vi "GEA2 Log Filter.vi"(1 "DST to ignore":string, 2 "Only print Dst":string, 5 "Filter Data":bool, 7 "GEA2 Msg":T1 {"Command" format="%02x"; "Destination" format="%02x"; "Source" format="%02x"}, 9 "Cmd to ignore":string, 11 "error in (no error)":errorcluster) -> (15 "error out":errorcluster)   [LabVIEW 2023]
uses:
  Common/LabVIEW GEA2 Toolkit/GEA3/type defs/Data In.ctl
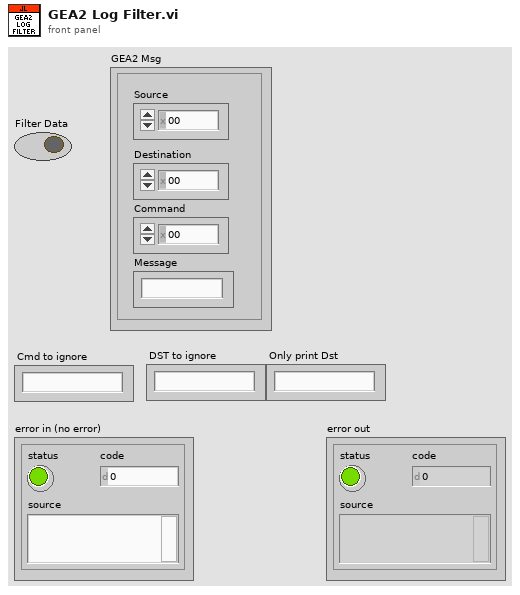
[diagram p1: front panel]
types:
  T1 = typedef "Data In.ctl" = cluster{"Source":u8, "Destination":u8, "Command":u8, "Message":string}
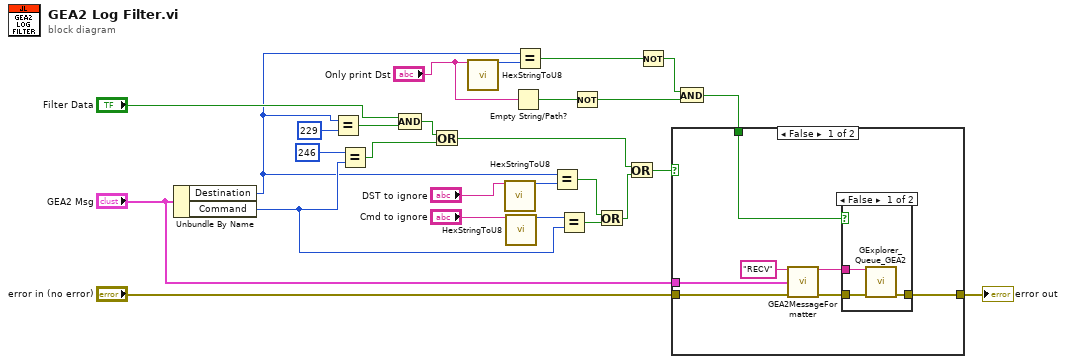
[diagram p0: block diagram]
diagram:
  n1 = Unbundle By Name("GEA2 Msg") -> ("Destination"=w7:u8, "Command"=w20:u8)
  n2 = Equal?(x=w7, y=u8 229) -> (x = y?=w26:bool)
  n3 = Equal?(x=u8 246 ("y"), y=w20) -> (x = y?=w19:bool)
  n4 = Compound Arithmetic op=AND("Filter Data", w26) -> (w18:bool)
  n5 = Or(x=w18, y=w19) -> (x .or. y?=w11:bool)
  n6 = call "HexStringToU8.vi"("Input String"="Only print Dst") -> ("Number Out"=w10:u8)  [unwired: 14 in]
  n7 = call "HexStringToU8.vi"("Input String"="DST to ignore") -> ("Number Out"=w14:u8)  [unwired: 14 in]
  n8 = call "HexStringToU8.vi"("Input String"="Cmd to ignore") -> ("Number Out"=w16:u8)  [unwired: 14 in]
  n9 = Empty String/Path?(string/path="Only print Dst") -> (empty?=w2:bool)
  n10 = Equal?(x=w7, y=w10) -> (x = y?=w6:bool)
  n11 = Equal?(x=w7, y=w14) -> (x = y?=w13:bool)
  n12 = Equal?(x=w16, y=w20) -> (x = y?=w15:bool)
  n13 = Not(x=w2) -> (.not. x?=w1:bool)
  n14 = Or(x=w13, y=w15) -> (x .or. y?=w12:bool)
  n15 = Or(x=w11, y=w12) -> (x .or. y?=w8:bool)
  n16 = Not(x=w6) -> (.not. x?=w4:bool)
  n17 = And(x=w4, y=w1) -> (x .and. y?=w3:bool)
  n18 = case shown="False" w8 {
    tunnel: "error in (no error)" -> [w34 w39]
    tunnel: "GEA2 Msg" -> [w33 _]
    tunnel: [w29 w39] -> w9
    tunnel: w3 -> [w28 _]
    frame False {
      n19 = call "GEA2MessageFormatter.vi"("Prefix(Send/Recv)"="RECV", "GEA2 Data In"=w33, "Error In"=w34) -> ("Output String"=w31:string, "Error Out"=w32:errorcluster)  [unwired: 11 in]
      n20 = case shown="False" w28 {
        tunnel: w32 -> [w37 w38]
        tunnel: [w36 w38] -> w29
        tunnel: w31 -> [w35 _]
        frame False {
          n21 = call "GExplorer_Queue_GEA2.vi"("Output String"=w35, "error in (no error)"=w37) -> ("error out"=w36:errorcluster)  [unwired: 13 in]
        }
        frame True {
        }
      }
    }
    frame True {
    }
  }
  "error out" <- w9
